vi "PWM.Measure.Analog.Convert.vi"(11 "Measurement":T2) -> (3 "Result":T1)   [LabVIEW 2018, in "Speciality FPGA IO.lvlib"]
uses:
  Speciality FPGA IO.lvlib
  Types/PWM.Measure.Analog.Measurement.ctl
  Types/PWM.Measure.Analog.Result.ctl
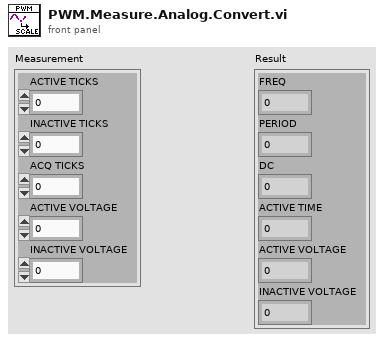
[diagram p1: front panel]
types:
  T1 = typedef "Speciality FPGA IO.lvlib/PWM.Measure.Analog.Result.ctl" = cluster{"FREQ":sgl, "PERIOD":sgl, "DC":sgl, "ACTIVE TIME":sgl, "ACTIVE VOLTAGE":sgl, "INACTIVE VOLTAGE":sgl}
  T2 = typedef "Speciality FPGA IO.lvlib/PWM.Measure.Analog.Measurement.ctl" = cluster{"ACTIVE TICKS":u32, "INACTIVE TICKS":u32, "ACQ TICKS":u32, "ACTIVE VOLTAGE":fxp<+/-,32,8>, "INACTIVE VOLTAGE":fxp<+/-,32,8>}
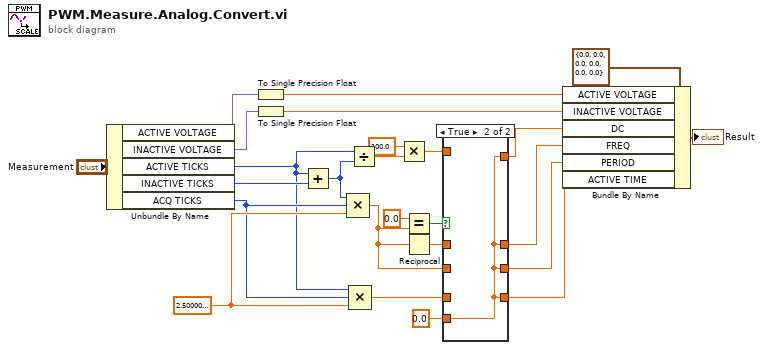
[diagram p0: block diagram]
diagram:
  w20 = sgl 2.5e-08 ("y")
  n1 = Unbundle By Name("Measurement") -> ("ACTIVE VOLTAGE"=w18:fxp<+/-,32,8>, "INACTIVE VOLTAGE"=w19:fxp<+/-,32,8>, "ACTIVE TICKS"=w3:u32, "INACTIVE TICKS"=w14:u32, "ACQ TICKS"=w12:u32)
  n2 = To Single Precision Float(number=w18) -> (single precision float=w6:sgl)
  n3 = To Single Precision Float(number=w19) -> (single precision float=w7:sgl)
  n4 = Add(x=w3, y=w14) -> (x+y=w22:u32)
  n5 = Compound Arithmetic op=MULTIPLY(w22, w12, w20) -> (w23:sgl)
  n6 = Divide(x=w3, y=w22) -> (x/y=w2:sgl)
  n7 = Compound Arithmetic op=MULTIPLY(w3, w12, w20) -> (w21:sgl)
  n8 = Multiply(x=sgl 100.0, y=w2) -> (x*y=w1:sgl)
  n9 = Equal?(x=sgl 0.0, y=w23) -> (x = y?=w17:bool)
  n10 = Reciprocal(x=w23) -> (1/x=w24:sgl)
  n11 = case shown="True" w17 {
    tunnel: [w26 w30] -> w9
    tunnel: [w27 w30] -> w8
    tunnel: [w29 w30] -> w10
    tunnel: w23 -> [w29 _]
    tunnel: [w28 w30] -> w11
    tunnel: w21 -> [w28 _]
    tunnel: w1 -> [w27 _]
    tunnel: w24 -> [w26 _]
    tunnel: sgl 0.0 ("x") -> [_ w30]
    frame False {
    }
    frame True {
    }
  }
  n12 = Bundle By Name(cluster=T1 {"FREQ"=0.0, "PERIOD"=0.0, "DC"=0.0, "ACTIVE TIME"=0.0, "ACTIVE VOLTAGE"=0.0, "INACTIVE VOLTAGE"=0.0} ("Analyzed"), "ACTIVE VOLTAGE"=w6, "INACTIVE VOLTAGE"=w7, "DC"=w8, "FREQ"=w9, "PERIOD"=w10, "ACTIVE TIME"=w11) -> (→"Result":T1)
